vi "watchPress_00.vi"() -> ()   [LabVIEW 2011]
panel:
  in  "stop":bool
  out "P(Torr)":string
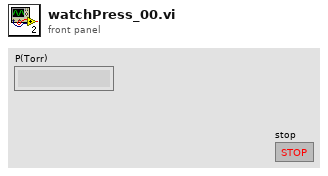
[diagram p1: front panel]
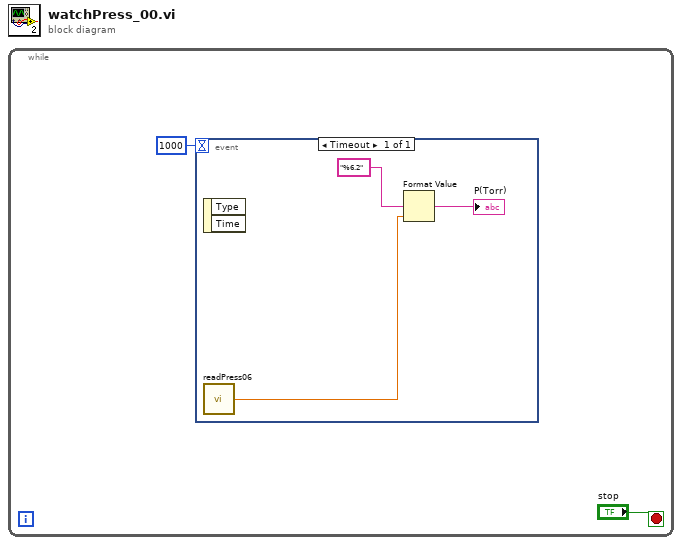
[diagram p0: block diagram]
diagram:
  n1 = while {
    stop <- "stop" stop-if-true
    n2 = event shown="[0] Timeout" {
      selector: _ -> [_]
      dyn-events: _ -> [_]
      timeout: 1000 -> [_]
      event Timeout {
        n3 = event-data() -> ()  [unwired: 1 in, 2 out]
        n4 = call "readPress06.vi"() -> ("P"=w4:dbl)
        n5 = Format Value(format string="%6.2", value (0)=w4) -> (output string=→"P(Torr)":string)  [unwired: 1 in]
      }
    }
  }
